vi "phase_write_txt.vi"(4 "Filename":string, 5 "Calibration folder":path, 8 "pixels":i32[](array[numeric]), 9 "wavelengths":dbl[](array[numeric]), 10 "voltages":dbl[](array[numeric]), 11 "phase":dbl[][](array[numeric])) -> (0 "error out":errorcluster, 1 "Boolean":bool, 2 "error?":bool, 3 "new file path (Not A Path if cancelled)":path)   [LabVIEW 2019]
uses:
  REFS.vi
  <vilib>/Utility/file.llb/Write Delimited Spreadsheet (DBL).vi
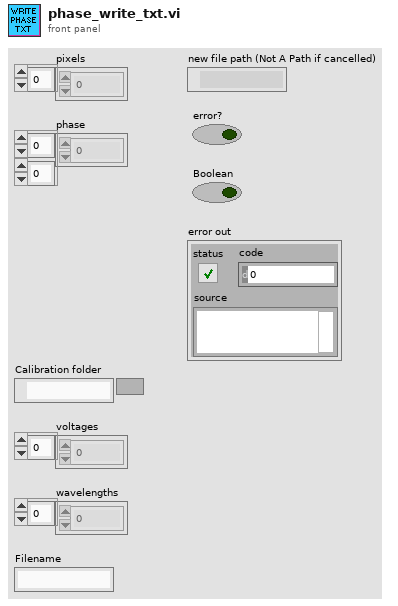
[diagram p1: front panel]
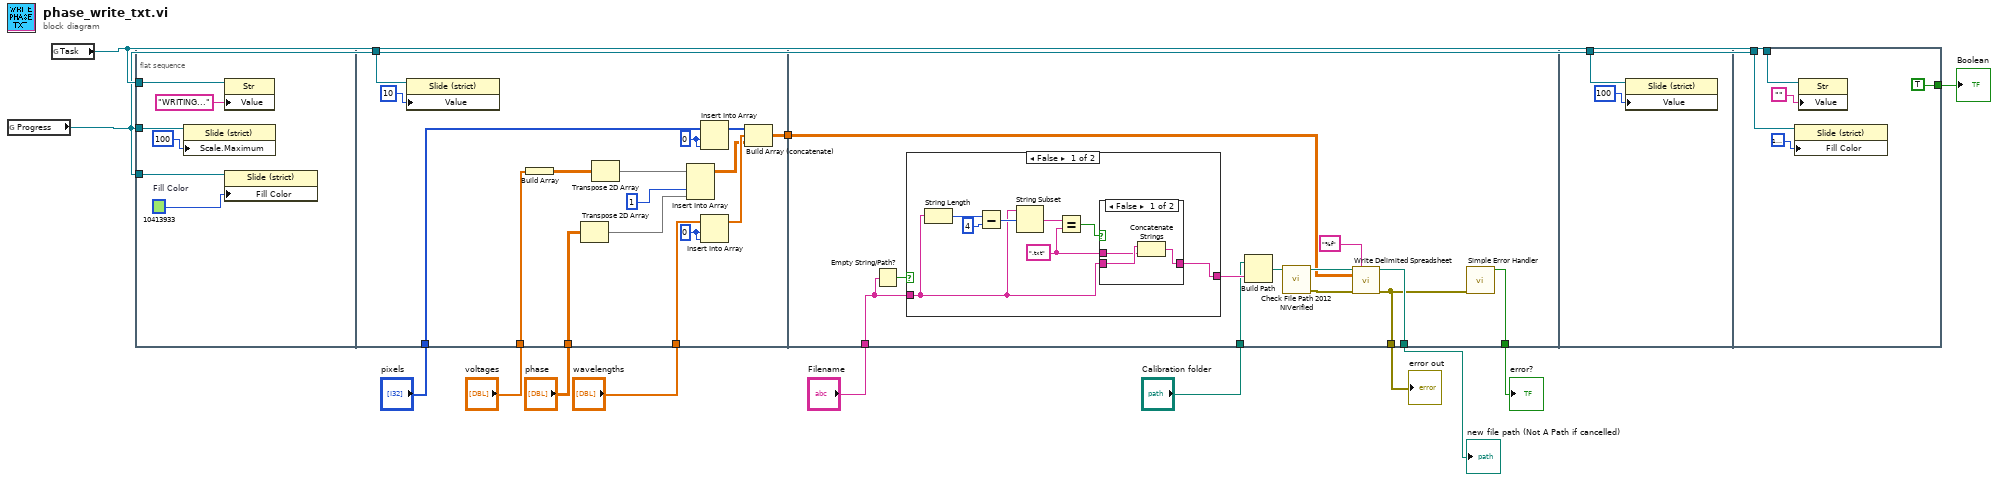
[diagram p0: block diagram]
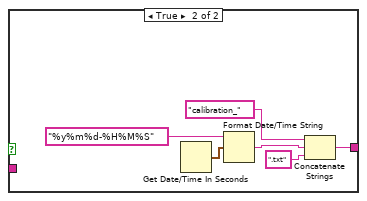
[diagram p3: hidden frame]
diagram:
  n1 = global read "REFS.vi" "Progress"() -> (w1:refnum<vi>)
  n2 = global read "REFS.vi" "Task"() -> (w2:refnum<vi>)
  n3 = flat-sequence {
    tunnel: w2 -> [w16]
    tunnel: w1 -> [w15]
    tunnel: w1 -> [w14]
    tunnel: "wavelengths" -> [w32]
    tunnel: "pixels" -> [w34]
    tunnel: "voltages" -> [w25]
    tunnel: "phase" -> [w24]
    tunnel: [w21] -> w13
    tunnel: w1 -> [w20]
    tunnel: w13 -> [w43]
    tunnel: "Filename" -> [w40]
    tunnel: "Calibration folder" -> [w39]
    tunnel: [w38] -> w10
    tunnel: [w37] -> w11
    tunnel: [w36] -> w12
    tunnel: w1 -> [w66]
    tunnel: [TRUE] -> w9
    tunnel: w1 -> [w69]
    tunnel: w2 -> [w68]
    frame #0 {
      w18 = u32 10413933  # Fill Color
      n4 = property on="Property Node" class="Slide (strict)"(reference=w14, "Scale.Maximum"=100) -> ()  [unwired: 1 in, 2 out]
      n5 = property class="Str"(reference=w16, "Value"="WRITING...") -> ()  [unwired: 1 in, 2 out]
      n6 = property on="Property Node" class="Slide (strict)"(reference=w15, "Fill Color"=w18) -> ()  [unwired: 1 in, 2 out]
    }
    frame #1 {
      w33 = 0 ("index")
      w35 = 0 ("index")
      n7 = property class="Slide (strict)"(reference=w20, "Value"=10) -> ()  [unwired: 1 in, 2 out]
      n8 = Build Array(w25) -> (w29:dbl[][])
      n9 = Transpose 2D Array(2D array=w24) -> (transposed array=w26:dbl[][])
      n10 = Transpose 2D Array(2D array=w29) -> (transposed array=w28:dbl[][])
      n11 = Insert Into Array(array=w28, index (col)=1, new element=w26) -> (w22:dbl[][])  [unwired: 1 in]
      n12 = Insert Into Array(array=w34, index=w35, new element=w35) -> (w31:i32[])
      n13 = Insert Into Array(array=w32, index=w33, new element=w33) -> (w30:dbl[])
      n14 = Build Array (concatenate)(w31, w30, w22) -> (w21:dbl[][])
    }
    frame #2 {
      n15 = Empty String/Path?(string/path=w40) -> (empty?=w47:bool)
      n16 = case shown="False" w47 {
        tunnel: w40 -> [w50 _]
        tunnel: [w49 w61] -> w46
        frame False {
          w48 = ".txt" ("y")
          n17 = String Length(string=w50) -> (length=w54:i32)
          n18 = Subtract(x=w54, y=4) -> (x-y=w55:i32)
          n19 = String Subset(string=w50, offset (0)=w55) -> (substring=w52:string)  [unwired: 1 in]
          n20 = Equal?(x=w52, y=w48) -> (x = y?=w51:bool)
          n21 = case shown="False" w51 {
            tunnel: [w57 w59] -> w49
            tunnel: w50 -> [w58 w59]
            tunnel: w48 -> [w56 _]
            frame False {
              n22 = Concatenate Strings(w58, w56) -> (w57:string)
            }
            frame True {
            }
          }
        }
        frame True {
          n23 = Get Date/Time In Seconds() -> (seconds since 1Jan1904=w65:timestamp)
          n24 = Format Date/Time String(time format string (%c)="%y%m%d-%H%M%S", seconds (now)=w65) -> (date/time string=w63:string)  [unwired: 1 in]
          n25 = Concatenate Strings("calibration_" ("string"), w63, ".txt" ("string")) -> (w61:string)
        }
      }
      n26 = Build Path(base path=w39, name or relative path=w46) -> (appended path=w45:path)
      n27 = call "Check File Path 2012 NIVerified.vi"("Path to Check"=w45) -> ("error out"=w41:errorcluster, "Valid Path"=w44:path)  [unwired: 7 in, 2 out]
      n28 = call-poly <vilib>:"Write Delimited Spreadsheet.vi"("file path (dialog if empty)"=w44, "format (%.3f)"="%f", "2D data"=w43, "error in (no error)"=w41) -> ("new file path (Not A Path if cancelled)"=w38:path, "error out"=w36:errorcluster)  [unwired: 10 in]
      n29 = call <vilib>:"Simple Error Handler.vi"("error in (no error)"=w36) -> ("error?"=w37:bool)  [unwired: 4 in, 4 out]
    }
    frame #3 {
      n30 = property class="Slide (strict)"(reference=w66, "Value"=100) -> ()  [unwired: 1 in, 2 out]
    }
    frame #4 {
      n31 = property on="Property Node" class="Slide (strict)"(reference=w69, "Fill Color"=u32 16777216) -> ()  [unwired: 1 in, 2 out]
      n32 = property class="Str"(reference=w68, "Value"="") -> ()  [unwired: 1 in, 2 out]
    }
  }
  "error out" <- w12
  "error?" <- w11
  "new file path (Not A Path if cancelled)" <- w10
  "Boolean" <- w9
